vi "create correspondence table.vi"(10 "pieces":i32, 11 "data array":sgl[][](array[numeric]) format="%.5f") -> (2 "calibration graph":cluster{dbl[], dbl[]}[](array[cluster]), 3 "correspondence table":T1 {"volts" format="%.4f"; "physical units" format="%.4f"})   [LabVIEW 2012]
doc: "Channel 0 in the data array is LDVT output converted to have units of length.\nChannel 1 in the data array is wave gage output in volts."
uses:
  correspondence table.ctl
  <vilib>/Analysis/baseanly.llb/Mean (DBL).vi
  <vilib>/Analysis/NI_AALPro.lvlib
  <vilib>/Analysis/NI_AALBase.lvlib
panel:
  # "physical"
  # "volts"
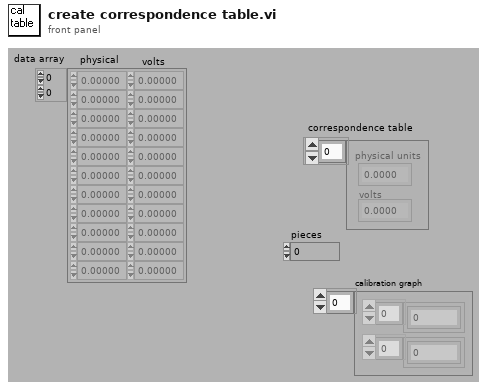
[diagram p1: front panel]
types:
  T1 = typedef "correspondence table.ctl" = cluster{"physical units":dbl, "volts":dbl}[]
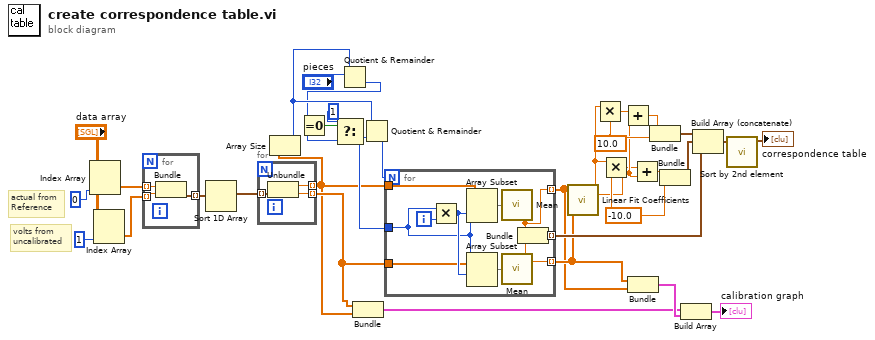
[diagram p0: block diagram]
diagram:
  w19 = 10.0
  w20 = -10.0
  # "actual from\nReference"
  # "volts from\nuncalibrated"
  n1 = Index Array(array="data array", index (col)=0 ("Index")) -> (element=w33:sgl[])  [unwired: 1 in]
  n2 = Index Array(array="data array", index (col)=1 ("Index")) -> (element=w31:sgl[])  [unwired: 1 in]
  n3 = for {
    tunnel: w33 -> [w37] mode=indexing
    tunnel: w31 -> [w36] mode=indexing
    tunnel: [w35] -> w30 mode=indexing
    n4 = Bundle(w37, w36) -> (w35:cluster{sgl, sgl})  [unwired: 1 in]
  }
  n5 = Sort 1D Array(array=w30) -> (sorted array=w29:cluster{sgl, sgl}[])
  n6 = for {
    tunnel: w29 -> [w40] mode=indexing
    tunnel: [w39] -> w3 mode=indexing
    tunnel: [w38] -> w4 mode=indexing
    n7 = Unbundle(w40) -> (w39:sgl, w38:sgl)
  }
  n8 = Array Size(array=w3) -> (size(s)=w28:i32)
  n9 = Quotient & Remainder(x=w28, y="pieces") -> (floor(x/y)=w24:i32)  [unwired: 1 out]
  n10 = Equal To 0?(x=w24) -> (x = 0?=w22:bool)
  n11 = Select(t=1, s=w22, f=w24) -> (s? t:f=w21:i32)
  n12 = Bundle(w4, w3) -> (w1:cluster{sgl[], sgl[]})  [unwired: 1 in]
  n13 = Quotient & Remainder(x=w28, y=w21) -> (floor(x/y)=w25:i32)  [unwired: 1 out]
  n14 = for {
    N: w25 -> [_]
    tunnel: w3 -> [w48]
    tunnel: w4 -> [w46]
    tunnel: [w43] -> w14 mode=indexing
    tunnel: w21 -> [w42]
    tunnel: [w41] -> w6 mode=indexing
    tunnel: [w44] -> w7 mode=indexing
    i -> [w50]
    n15 = Multiply(x=w42, y=w50) -> (x*y=w47:i32)
    n16 = Array Subset(array=w48, index=w47, length=w42) -> (w49:sgl[])
    n17 = Array Subset(array=w46, index=w47, length=w42) -> (w45:sgl[])
    n18 = call-poly <vilib>:"Mean.vi"("X"=w49) -> ("mean"=w41:dbl)  [unwired: 1 out]
    n19 = call-poly <vilib>:"Mean.vi"("X"=w45) -> ("mean"=w44:dbl)  [unwired: 1 out]
    n20 = Bundle("mean"=w41, "mean"=w44) -> (w43:cluster{"mean":dbl, "mean":dbl})  [unwired: 1 in]
  }
  n21 = call <vilib>:"Linear Fit Coefficients.vi"("Y"=w6, "X"=w7) -> ("slope"=w9:dbl, "intercept"=w10:dbl)  [unwired: 11 in, 1 out]
  n22 = Multiply(x=w9, y=w19) -> (x*y=w18:dbl)
  n23 = Multiply(x=w9, y=w20) -> (x*y=w8:dbl)
  n24 = Add(x=w18, y=w10) -> (x+y=w17:dbl)
  n25 = Bundle(w7, w6) -> (w2:cluster{dbl[], dbl[]})  [unwired: 1 in]
  n26 = Add(x=w8, y=w10) -> (x+y=w11:dbl)
  n27 = Bundle(w17, w19) -> (w16:cluster{dbl, dbl})  [unwired: 1 in]
  n28 = Bundle(w11, w20) -> (w15:cluster{dbl, dbl})  [unwired: 1 in]
  n29 = Build Array(w1, w2) -> (→"calibration graph":cluster{dbl[], dbl[]}[])
  n30 = Build Array (concatenate)(w16, w15, w14) -> (w13:cluster{"mean":dbl, "mean":dbl}[])
  n31 = call "Sort by 2nd element.vi"("correspondence table in"=w13) -> ("correspondence table out"=→"correspondence table":T1)  [unwired: 9 in]
